vi "kill broken bundle.vi"(8 "error in":errorcluster, 11 "VI in":refnum<vi>) -> (0 "error out":errorcluster, 3 "reference out":refnum<vi>)   [LabVIEW 2013, in "scripting tools.lvlib"]
uses:
  <vilib>/Utility/traverseref.llb/TRef TravTarget.ctl
  scripting tools.lvlib
  <vilib>/Utility/traverseref.llb/VI Scripting - Traverse.lvlib
  <vilib>/Utility/VariantDataType/VariantType.lvlib
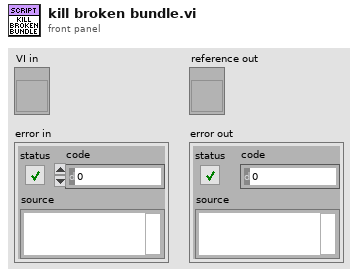
[diagram p1: front panel]
types:
  T1 = typedef "TRef TravTarget.ctl" = enum16{"FP", "BD", "Other"}
  T2 = typedef "VariantType.lvlib/Type.ctl" = enum8{"Invalid Type", "Void", "I8", "I16", "I32", "I64", "U8", "U16", "U32", "U64", "Single Float", "Double Float", "Extended Float", "Single Complex", "Double Complex", "Extended Complex", "Enum U8", "Enum U16", "Enum U32", "Enum U64", "Single Float With Unit", "Double Float With Unit", "Extended Float With Unit", "Single Complex with Unit", "Double Complex with Unit", "Extended Complex with Unit", "Boolean", "String", "Path", "Picture", "Tag", "Array", "Cluster", "Variant", "LV Variant", "Waveform", "Timestamp", "Digital Waveform", "Digital Data", "ExpressData", "Refnum", "External Data", "VI", "Poly VI", "LabVIEW Class Instance", "Fixed Point"}
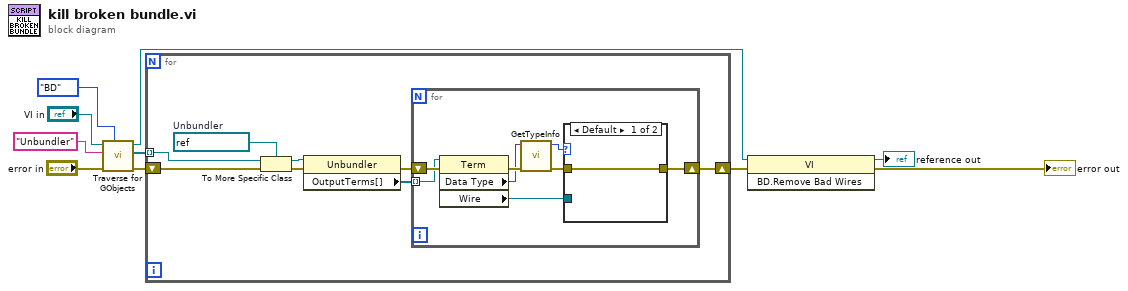
[diagram p0: block diagram]
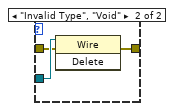
[diagram p2: hidden frame]
diagram:
  n1 = call <vilib>:"Traverse for GObjects.vi"("Traverse Target"=TRef_TravTarget."BD", "error in (no error)"="error in", "Class Name"="Unbundler", "VI Refnum"="VI in") -> ("error out"=w7:errorcluster, "References"=w6:refnum<vi>[], "dup VI Refnum"=w4:refnum<vi>)  [unwired: 4 in, 1 out]
  n2 = for {
    shift-right: [w12] -> w5
    shift-left: w7 -> [w17]
    tunnel: w6 -> [w16] mode=indexing
    w18 = refnum<vi> refnum  # Unbundler
    n3 = To More Specific Class(target class=w18, reference=w16, error in=w17) -> (specific class reference=w15:refnum<vi>, error out=w14:errorcluster)
    n4 = property class="Unbundler"(reference=w15, error in=w14) -> (error out=w13:errorcluster, "OutputTerms[]"=w11:refnum<vi>[])  [unwired: 1 out]
    n5 = for {
      shift-right: [w25] -> w12
      shift-left: w13 -> [w26]
      tunnel: w11 -> [w19] mode=indexing
      n6 = property class="Term"(reference=w19, error in=w26) -> (error out=w24:errorcluster, "Data Type"=w20:variant, "Wire"=w23:refnum<vi>)  [unwired: 1 out]
      n7 = call <vilib>:"GetTypeInfo.vi"("error in (no error)"=w24, "Variant"=w20) -> ("error out"=w22:errorcluster, "Type Enum"=w21:T2)  [unwired: 5 in, 3 out]
      n8 = case shown="Default" w21 {
        tunnel: [w27 w30] -> w25
        tunnel: w23 -> [_ w29]
        tunnel: w22 -> [w27 w28]
        frame Default {
        }
        frame "Invalid Type", "Void" {
          n9 = invoke class="Wire" method="Delete"(reference=w29, error in=w28) -> (error out=w30:errorcluster)  [unwired: 1 in, 2 out]
        }
      }
    }
  }
  n10 = invoke class="VI" method="BD.Remove Bad Wires"(reference=w4, error in=w5) -> (reference out=→"reference out":refnum<vi>, error out=→"error out":errorcluster)  [unwired: 1 in, 1 out]
